vi "Write pubSubDataEvent.vi"(10 "pubSubDataEvent":refnum<class "PubSubDataEvent.lvclass">, 11 "MiddlewareSVThisComponent in":refnum<class "MiddlewareSVThisComponent.lvclass">) -> (3 "MiddlewareSVThisComponent out":refnum<class "MiddlewareSVThisComponent.lvclass">)   [LabVIEW 2015, in "MiddlewareSVThisComponent.lvclass"]
uses:
  MiddlewareSVThisComponent.lvclass
  PubSubDataEvent/PubSubDataEvent.lvclass
  MiddlewareSVThisComponent.lvclass/MiddlewareSVThisComponent.ctl
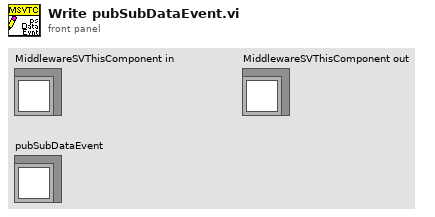
[diagram p1: front panel]
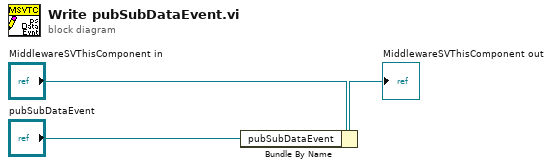
[diagram p0: block diagram]
diagram:
  n1 = Bundle By Name(cluster="MiddlewareSVThisComponent in", "pubSubDataEvent"="pubSubDataEvent") -> (→"MiddlewareSVThisComponent out":refnum<class "MiddlewareSVThisComponent.lvclass">)
